vi "Add Without Dup Priv.vi"(4 "Add String":string, 5 "Strings In":string[](array[string])) -> (2 "Strings Out":string[](array[string]))   [LabVIEW 2017, in "Tree API.lvlib" / "Tree.lvclass"]
uses:
  Tree.lvclass
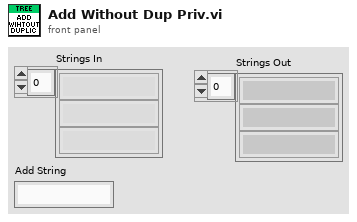
[diagram p1: front panel]
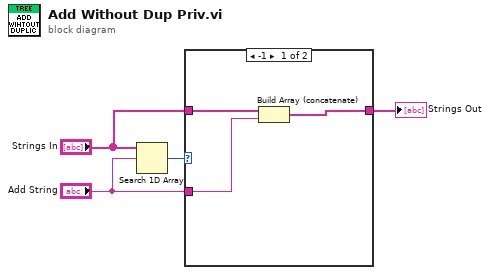
[diagram p0: block diagram]
diagram:
  n1 = Search 1D Array(1D array="Strings In", element="Add String") -> (index of element=w4:i32)  [unwired: 1 in]
  n2 = case shown="-1" w4 {
    tunnel: "Strings In" -> [w7 w8]
    tunnel: "Add String" -> [w6 _]
    tunnel: [w5 w8] -> w1
    frame -1 {
      n3 = Build Array (concatenate)(w7, w6) -> (w5:string[])
    }
    frame Default {
    }
  }
  "Strings Out" <- w1
